vi "Enable Close Inlet.vi"(0 "FPGA API in":refnum<class "FPGA API Mock.lvclass">, 11 "error in (no error)":errorcluster, 13 "Direction":T1=enum."Chamber") -> (4 "FPGA API out":refnum<class "FPGA API Mock.lvclass">, 15 "error out":errorcluster)   [LabVIEW 2019, in "FPGA API Mock.lvclass"]
uses:
  FPGA API Mock.lvclass
  TypeDef/Direction.ctl
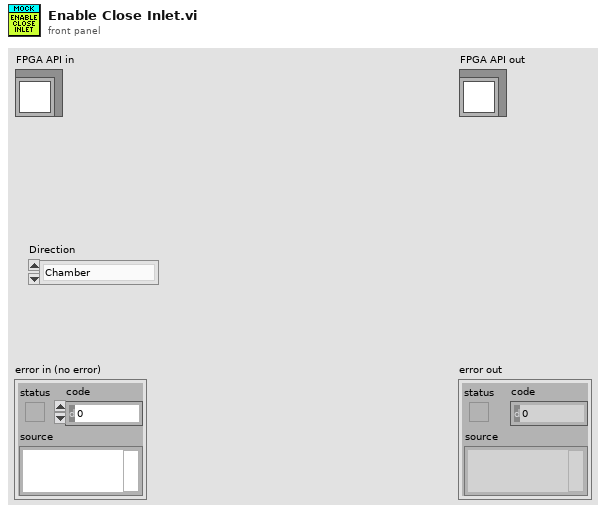
[diagram p1: front panel]
types:
  T1 = typedef "Direction.ctl" = enum16{"None", "Chamber", "DUT"}
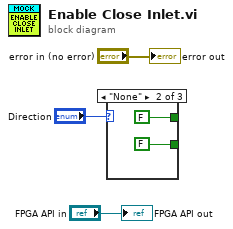
[diagram p0: block diagram]
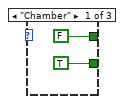
[diagram p2: hidden frame]
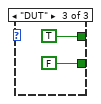
[diagram p3: hidden frame]
diagram:
  n1 = case shown="\"None\"" "Direction" {
    tunnel: [FALSE ("Enable Close Inlet") FALSE ("Enable Close Inlet") TRUE ("Enable Close Inlet")] -> _
    tunnel: [TRUE ("Enable Close Inlet") FALSE ("Enable Close Inlet") FALSE ("Enable Close Inlet")] -> _
    frame "Chamber" {
    }
    frame "None" {
    }
    frame "DUT" {
    }
  }
  "error out" <- "error in (no error)"
  "FPGA API out" <- "FPGA API in"
